vi "Scroll Right.vi"(8 "error in (no error)":errorcluster, 10 "VISA resource name in":refnum<visa-resource-name>, 11 "LCD-I2C in":refnum<class "LCD-I2C.lvclass">) -> (0 "error out":errorcluster, 2 "VISA resource name":refnum<visa-resource-name>, 3 "LCD-I2C out":refnum<class "LCD-I2C.lvclass">)   [LabVIEW 2023, in "CTI-Visa-DeviceLib.lvlib" / "LCD-I2C.lvclass"]
uses:
  LCD-I2C.lvclass
  LCD-I2C.lvclass/LCD-I2C.ctl
  Command.ctl
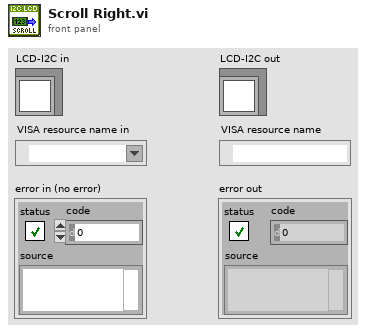
[diagram p1: front panel]
types:
  T1 = typedef "CTI-Visa-DeviceLib.lvlib/LCD-I2C.lvclass/Command.ctl" = enum16{"Clear Display", "Return Home", "Entry Mode Set", "Display Control", "Cursor Shift", "Function Set", "Set CGRAM Addr", "Set DDRAM Addr"}
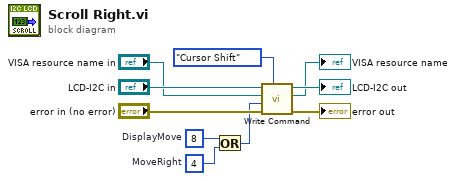
[diagram p0: block diagram]
diagram:
  w1 = u8 4  # MoveRight
  w3 = u8 8  # DisplayMove
  n1 = Or(x=w3, y=w1) -> (x .or. y?=w2:u8)
  n2 = call "Write Command.vi"("Command"=Command."Cursor Shift", "error in (no error)"="error in (no error)", "Value"=w2, "VISA resource name in"="VISA resource name in", "LCD-I2C in"="LCD-I2C in") -> ("error out"=→"error out":errorcluster, "VISA resource name"=→"VISA resource name":refnum<visa-resource-name>, "LCD-I2C out"=→"LCD-I2C out":refnum<class "LCD-I2C.lvclass">)  [unwired: 4 in]
